vi "Enqueue Multiple Messages.vi"(8 "data array":variant[](array[variant]), 11 "cmd array":string[](array[string])) -> (3 "channel":T1)   [LabVIEW 2023, in "Message Queue.lvlib"]
doc: "This VI puts messages into the messenger channel."
uses:
  Message Queue.lvlib
  <extravilib>/ChannelInstances/Messenger-t'Message Queue.lvlib-Message Cluster.ctl'/))Channel.ctl
  Message Cluster.ctl
  <extravilib>/ChannelInstances/Messenger-t'Message Queue.lvlib-Message Cluster.ctl'/Write With Abort.vi
  <extravilib>/ChannelInstances/Messenger-t'Message Queue.lvlib-Message Cluster.ctl'/Endpoint.vi
  <extravilib>/ChannelInstances/Messenger-t'Message Queue.lvlib-Message Cluster.ctl'.lvlib
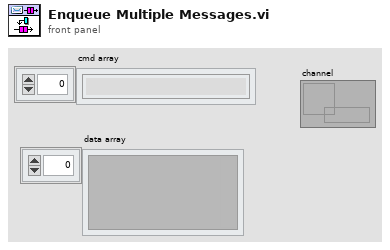
[diagram p1: front panel]
types:
  T1 = typedef "Messenger-t'Message Queue.lvlib-Message Cluster.ctl'.lvlib/))Channel.ctl" = refnum<queue>
  T2 = typedef "Message Queue.lvlib/Message Cluster.ctl" = cluster{"Message":string, "Message Data":variant}
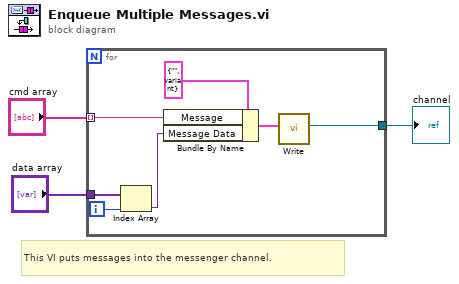
[diagram p0: block diagram]
diagram:
  # "This VI puts messages into the messenger channel."
  n1 = for {
    tunnel: "cmd array" -> [w8] mode=indexing
    tunnel: "data array" -> [w6]
    tunnel: [w4] -> w1
    i -> [w7]
    n2 = Index Array(array=w6, index=w7) -> (element=w5:variant)
    n3 = Bundle By Name(cluster=T2 {"Message"="", "Message Data"=variant} ("Message Cluster"), "Message"=w8, "Message Data"=w5) -> (w9:T2)
    n4 = call <extravilib>:"Write.vi"("element"=w9) -> ("channel"=w4:T1)  [unwired: 8 in, 2 out]
  }
  "channel" <- w1
